vi "SVPO Power Spectrum (1 Ch DBL Array).vi"(0 "scaled signal [EU]":dbl[](array[numeric]), 1 "sampling rate [Hz]":dbl=1.0, 2 "window":T7=1 items=["None"=0, "Hanning"=1, "Hamming"=2, "Blackman-Harris"=3, "Exact Blackman"=4, "Blackman"=5, "Flat Top"=6, "4 Term B-Harris "=7, "7 Term B-Harris"=8, "Low Sidelobe"=9, "Force"=64, "Exponential"=65, "Blackman Nuttall"=11, "Triangle"=30, "Bartlett-Hanning"=31, "Bohman"=32, "Parzen"=33, "Welch"=34, "Kaiser"=60, "Dolph-Chebyshev"=61, "Gaussian"=62], 9 "restart averaging? (F)":bool) -> (13 "averages completed":dbl, 14 "power spectrum [EU^2 rms]":cluster{"f0":dbl, "df":dbl, "magnitude":dbl[]} {"magnitude" format="%.2p"; "df" format="%.2p"; "f0" format="%.2p"}, 18 "spectrum info":T1={"channel name"="", "description"="", "x-axis units"=0, "spectral info"={"spectrum type"=enum."Power [Magnitude^2]", "linear/dB"=enum."linear", "window"=0, "window size"=0, "FFT size"=0}, "engineering units"=0, "custom label"="", "dB reference [EU]"=0.0, "peak units"=enum."rms", "weighting filter"=0, "spectral density?"=FALSE, "unit label"="", "spectrum skewed?"=FALSE, "complimentary spectrum units"=enum."none"} {"x-axis units" items=["Time (s)"=0, "Frequency-CB (Hz)"=1, "Frequency-CPB (Hz)"=1248, "Frequency-Arbitrary (Hz)"=2357, "Quefrency (s)"=2, "Revolutions (rev)"=3, "Order"=4, "Speed (RPM)"=11, "Speed (rad/s)"=21, "Index"=65535]; "weighting filter" items=["Linear", "A-weighting", "B-weighting", "C-weighting", "ITU-R 468-4", "Dolby", "CCITT", "C-message", "Wb", "Wc", "Wd", "We", "Wf", "Wh", "Wj", "Wk", "Wm", "AES17 20 kHz lowpass", "AES17 40 kHz lowpass", "AES17 20 kHz highpass", "AES17 40 kHz highpass"]; "dB reference [EU]" format="%.2f"; "engineering units" items=["custom..."=0, "V"=1, "A"=21, "C"=30, "pC"=31, "s"=32, "-"=29, "Pa"=2, "N"=20, "g"=3, "m/s^2"=4, "m/s"=5, "m"=6, "mm/s"=12, "mm"=13, "micron/s"=14, "micron"=15, "in/s^2"=7, "in/s"=8, "in"=9, "mil/s"=10, "mil"=11, "rad/s^2"=16, "rad/s"=17, "rad"=18, "deg/s^2"=26, "deg/s"=27, "deg"=28, "RPM"=22, "cycle/s^2"=23, "Hz"=24, "cycle"=25, "strain"=19]; "spectral info"."window" items=["None "=0, "Hanning"=1, "Hamming"=2, "Blackman-Harris"=3, "Exact Blackman"=4, "Blackman"=5, "Flat Top"=6, "4 Term B-Harris "=7, "7 Term B-Harris"=8, "Low Sidelobe"=9, "Force - Exponential"=10, "Gaussian"=62]})   [LabVIEW 2017]
doc: "Computes the linear RMS-averaged power spectrum of <B>scaled signal [EU]</B> in a linear scale. Use the power spectrum to quantify signal components as a function of frequency. Use this VI on embedded targets that have limited computational resources. Wire data to the <B>scaled signal [EU]</B> input to determine the polymorphic instance to use or manually select the instance."
uses:
  <vilib>/addons/_NISVFA/_Shared subVIs/Controls/svc_Window.ctl
  <vilib>/addons/_NISVFA/_Shared subVIs/Controls/svc_Spectrum Info.ctl
  <vilib>/addons/_NISVFA/_Shared subVIs/Controls/svc_X-Axis Units.ctl
  <vilib>/addons/_NISVFA/_Shared subVIs/Controls/svc_Spectrum Type.ctl
  <vilib>/addons/_NISVFA/_Shared subVIs/Controls/svc_Engineering Units Text Ring.ctl
  <vilib>/addons/_NISVFA/_Shared subVIs/Controls/svc_Weighting Filter Text Ring.ctl
  <vilib>/addons/_NISVFA/_Shared subVIs/Controls/svc_Complimentary Spectrum Units.ctl
  <vilib>/Analysis/2dsp.llb/Power Spectrum (DBL).vi
  <vilib>/Analysis/4window.llb/Force Window.vi
  <vilib>/Analysis/4window.llb/Force Window (DBL).vi
  <vilib>/Analysis/4window.llb/Exponential Window.vi
  <vilib>/Analysis/4window.llb/Exponential Window (DBL).vi
  <vilib>/Utility/error.llb/Error Cluster From Error Code.vi
  <vilib>/Analysis/0measdsp.llb/Scaled Time Domain Window.vi
  <vilib>/Analysis/0measdsp.llb/Scaled Time Domain Window (DBL).vi
  <vilib>/addons/_NISVFA/_Spectrum Processing/subVIs/svfa_Spectrum Info Window to windowTd Type Def.vi
  <vilib>/Analysis/NI_AALPro.lvlib
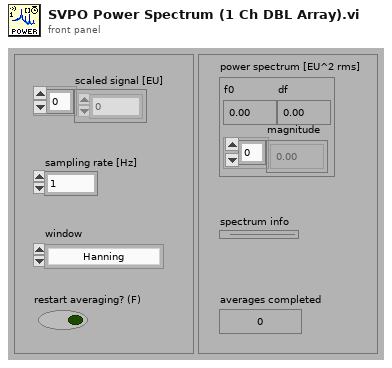
[diagram p1: front panel]
types:
  T1 = typedef "svc_Spectrum Info.ctl" = cluster{"channel name":string, "description":string, "x-axis units":T2, "spectral info":cluster{"spectrum type":T3, "linear/dB":enum16{"linear", "dB"}, "window":u16, "window size":i32, "FFT size":i32}, "engineering units":T4, "custom label":string, "dB reference [EU]":dbl, "peak units":enum16{"rms", "peak", "peak-peak"}, "weighting filter":T5, "spectral density?":bool, "unit label":string, "spectrum skewed?":bool, "complimentary spectrum units":T6}
  T2 = typedef "svc_X-Axis Units.ctl" = u16
  T3 = typedef "svc_Spectrum Type.ctl" = enum16{"FFT Spectrum [complex]", "Amplitude [Magnitude]", "Power [Magnitude^2]", "Cross Spectrum [complex]", "Frequency Response [Complex]"}
  T4 = typedef "svc_Engineering Units Text Ring.ctl" = u16
  T5 = typedef "svc_Weighting Filter Text Ring.ctl" = u16
  T6 = typedef "svc_Complimentary Spectrum Units.ctl" = enum16{"none", "radians", "degrees", "cycles", "imaginary"}
  T7 = typedef "svc_Window.ctl" = u32
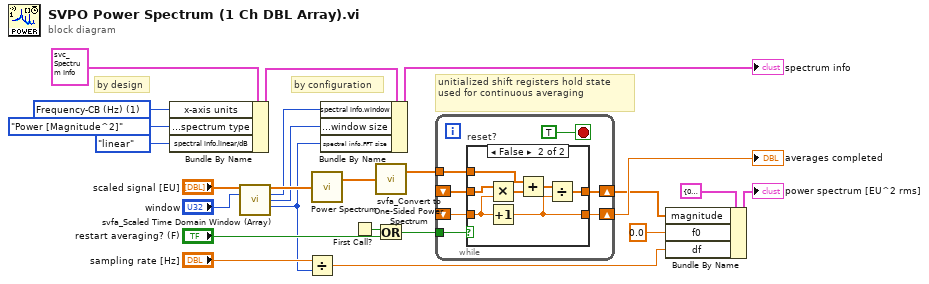
[diagram p0: block diagram]
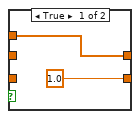
[diagram p2: hidden frame]
diagram:
  w3 = T2 1 items=["Time (s)"=0, "Frequency-CB (Hz)"=1, "Frequency-CPB (Hz)"=1248, "Frequency-Arbitrary (Hz)"=2357, "Quefrency (s)"=2, "Revolutions (rev)"=3, "Order"=4, "Speed (RPM)"=11, "Speed (rad/s)"=21, "Critical Band"=31, "Critical Band Rate (Bark)"=32, "Index"=65535] ("x-axis units")
  # "unitialized shift registers hold state used for continuous averaging"
  # "by configuration"
  # "by design"
  n1 = Bundle By Name(cluster=T1 {"channel name"="", "description"="", "x-axis units"=1, "spectral info"={"spectrum type"=enum."Power [Magnitude^2]", "linear/dB"=enum."linear", "window"=0, "window size"=0, "FFT size"=0}, "engineering units"=0, "custom label"="EU", "dB reference [EU]"=0.0, "peak units"=enum."rms", "weighting filter"=0, "spectral density?"=FALSE, "unit label"="", "spectrum skewed?"=FALSE, "complimentary spectrum units"=enum."none"} ("spectrum info in"), "x-axis units"=w3, "spectral info.spectrum type"=svc_Spectrum_Type."Power [Magnitude^2]" ("spectrum type"), "spectral info.linear/dB"=enum16{"linear", "dB"}."linear" ("linear/dB")) -> (w4:T1)
  n2 = call <vilib>:"svfa_Scaled Time Domain Window (Array).vi"("input signal"="scaled signal [EU]", "window"="window") -> ("windowed signal"=w17:dbl[], "dup window"=w15:T7, "window length"=w14:i32, "FFT length"=w16:i32)  [unwired: 8 in, 2 out]
  n3 = Divide(x="sampling rate [Hz]", y=w16) -> (x/y=w9:dbl)
  n4 = call-poly <vilib>:"Power Spectrum.vi"("X"=w17) -> ("Power Spectrum"=w18:dbl[])  [unwired: 1 out]
  n5 = Bundle By Name(cluster=w4, "spectral info.window"=w15, "spectral info.window size"=w14, "spectral info.FFT size"=w16) -> (→"spectrum info":T1)
  n6 = First Call?() -> (First Call?: T/F=w20:bool)
  n7 = call <vilib>:"svfa_Convert to One-Sided Power Spectrum.vi"("two-sided power spectrum"=w18) -> ("one-sided power spectrum"=w19:dbl[])  [unwired: 1 out]
  n8 = Or(x=w20, y="restart averaging? (F)") -> (x .or. y?=w13:bool)
  n9 = while {
    tunnel: w13 -> [w27]
    shift-right: [w30] -> w12
    shift-left: _ -> [w28]
    shift-right: [w25] -> w8
    shift-left: _ -> [w29]
    tunnel: w19 -> [w26]
    stop <- TRUE stop-if-true
    n10 = case "reset?" shown="False" w27 {
      tunnel: [w32 w36] -> w25
      tunnel: [1.0 ("f0") w38] -> w30
      tunnel: w29 -> [_ w34]
      tunnel: w28 -> [_ w37]
      tunnel: w26 -> [w32 w35]
      frame True {
      }
      frame False {
        n11 = Multiply(x=w34, y=w37) -> (x*y=w40:dbl[])
        n12 = Increment(x=w37) -> (x+1=w38:dbl)
        n13 = Add(x=w35, y=w40) -> (x+y=w39:dbl[])
        n14 = Divide(x=w39, y=w38) -> (x/y=w36:dbl[])
      }
    }
  }
  "averages completed" <- w12
  n15 = Bundle By Name(cluster=cluster{"f0":dbl, "df":dbl, "magnitude":dbl[]} {"f0"=0.0, "df"=0.0, "magnitude"=[]} ("power spectrum [EU] 2"), "magnitude"=w8, "f0"=0.0, "df"=w9) -> (→"power spectrum [EU^2 rms]":cluster{"f0":dbl, "df":dbl, "magnitude":dbl[]})
